vi "Get_Fluid_Properties.vi"(4 "Fluid Properties":T3) -> (1 "Thermo and Transport Properties":T1)   [LabVIEW 2011]
uses:
  fluid_types.ctl
  fluid_properties.ctl
  <vilib>/gmath/interp.llb/Create Mesh Grid (2D) (x,y arrays).vi
  <vilib>/Utility/file.llb/Read From Spreadsheet File (DBL).vi
  <vilib>/gmath/interp.llb/Interpolate 2D (2d X,Y).vi
  <vilib>/gmath/NI_Gmath.lvlib
panel:
  out "Data":dbl[][][](array[numeric])
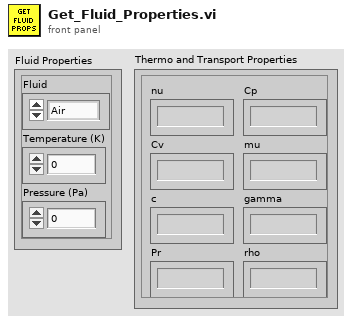
[diagram p1: front panel]
types:
  T1 = typedef "fluid_properties.ctl" = cluster{"nu":dbl, "c":dbl, "Pr":dbl, "Cp":dbl, "Cv":dbl, "gamma":dbl, "mu":dbl, "rho":dbl}
  T2 = typedef "fluid_types.ctl" = enum16{"Air", "Water"}
  T3 = cluster{"Fluid":T2, "Temperature (K)":dbl, "Pressure (Pa)":dbl}
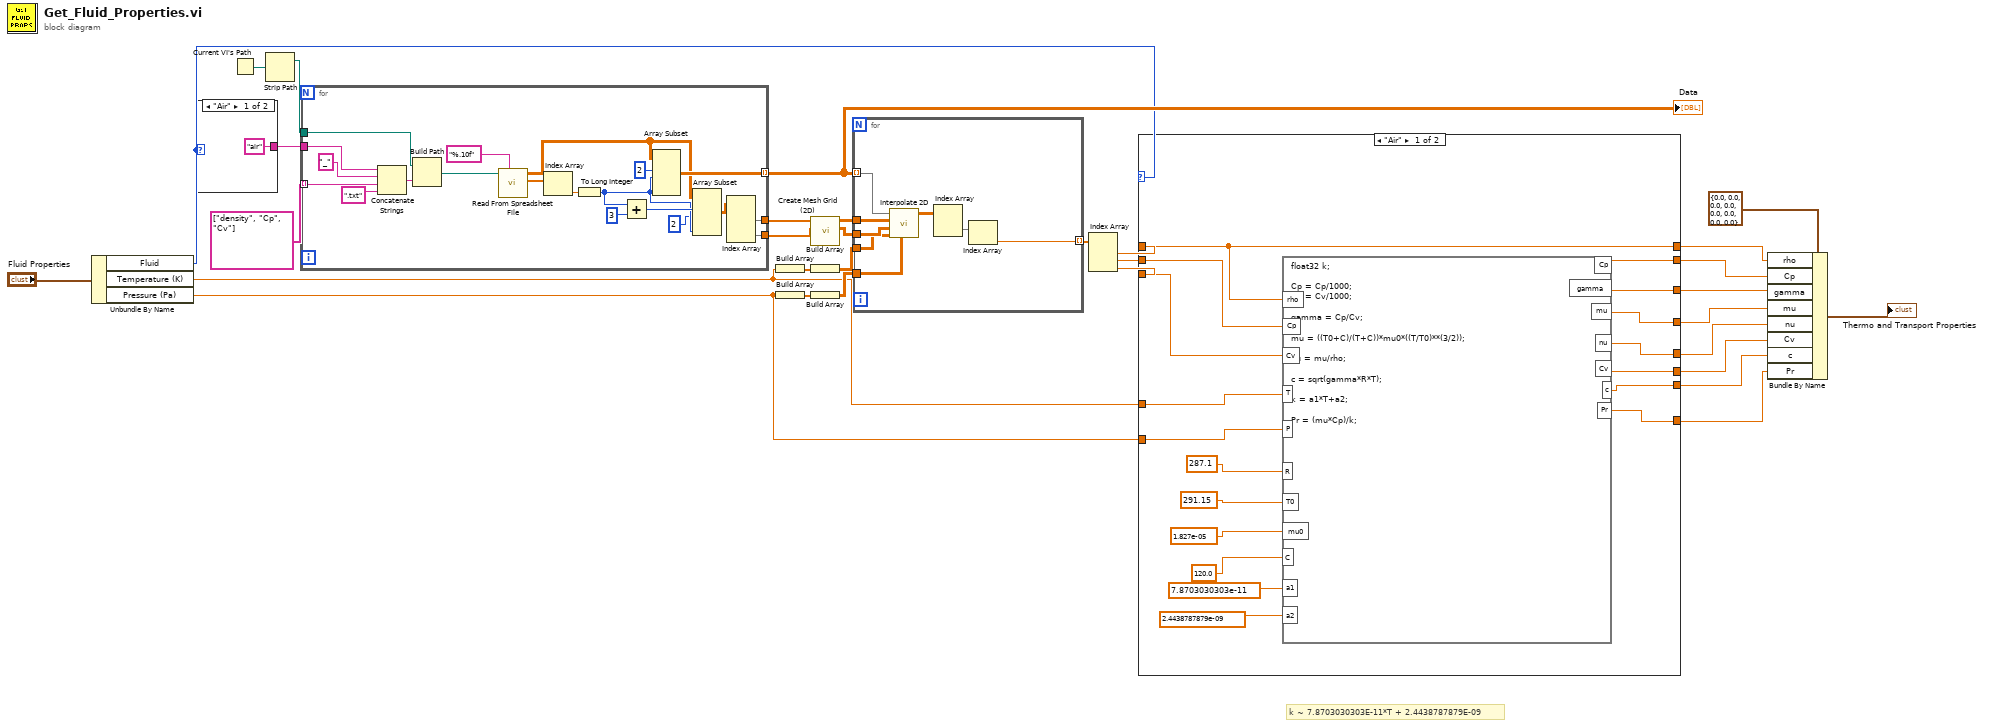
[diagram p0: block diagram]
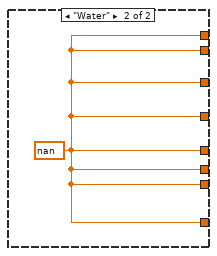
[diagram p2: hidden frame]
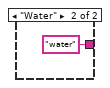
[diagram p3: hidden frame]
diagram:
  # "k ~ 7.8703030303E-11*T + 2.4438787879E-09"
  n1 = Unbundle By Name("Fluid Properties") -> ("Fluid"=w11:T2, "Temperature (K)"=w12:dbl, "Pressure (Pa)"=w13:dbl)
  n2 = case shown="\"Air\"" w11 {
    tunnel: ["air" "water"] -> w30
    frame "Air" {
    }
    frame "Water" {
    }
  }
  n3 = Current VI's Path() -> (path=w29:path)
  n4 = Strip Path(path=w29) -> (stripped path=w27:path)  [unwired: 1 out]
  n5 = for {
    tunnel: w30 -> [w52]
    tunnel: string[] ["density", "Cp", "Cv"] -> [w50] mode=indexing
    tunnel: w27 -> [w53]
    tunnel: [w44] -> w24 mode=indexing
    tunnel: [w35] -> w25
    tunnel: [w34] -> w26
    n6 = Concatenate Strings(w52, "_" ("string"), w50, ".txt" ("string")) -> (w48:string)
    n7 = Build Path(base path=w53, name or relative path=w48) -> (appended path=w47:path)
    n8 = call-poly <vilib>:"Read From Spreadsheet File.vi"("format (%.3f)"="%.10f", "file path (dialog if empty)"=w47) -> ("first row"=w45:dbl[], "all rows"=w41:dbl[][])  [unwired: 5 in, 3 out]
    n9 = Index Array(array=w45) -> (element=w43:dbl)  [unwired: 1 in]
    n10 = To Long Integer(number=w43) -> (32bit integer=w38:i32)
    n11 = Add(x=w38, y=3) -> (x+y=w39:i32)
    n12 = Array Subset(array=w41, index (row)=2 ("index"), length (row)=w38, length (col)=w38) -> (w44:dbl[][])  [unwired: 1 in]
    n13 = Array Subset(array=w41, index (row)=w39, length (row)=2 ("length"), length (col)=w38) -> (w36:dbl[][])  [unwired: 1 in]
    n14 = Index Array(array=w36) -> (element #1=w34:dbl[], element #2=w35:dbl[])  [unwired: 4 in]
  }
  "Data" <- w24
  n15 = Build Array(w12) -> (w20:dbl[])
  n16 = Build Array(w13) -> (w18:dbl[])
  n17 = call-poly <vilib>:"Create Mesh Grid (2D).vi"("y domain"=w25, "x domain"=w26) -> ("Y"=w22:dbl[][], "X"=w23:dbl[][])  [unwired: 7 in, 1 out]
  n18 = Build Array(w20) -> (w21:dbl[][])
  n19 = Build Array(w18) -> (w19:dbl[][])
  n20 = for {
    tunnel: w24 -> [w61] mode=indexing
    tunnel: w23 -> [w60]
    tunnel: w22 -> [w59]
    tunnel: w21 -> [w58]
    tunnel: w19 -> [w57]
    tunnel: [w54] -> w17 mode=indexing
    n21 = call-poly <vilib>:"Interpolate 2D.vi"("yi"=w57, "xi"=w58, "Y"=w59, "X"=w60, "Z"=w61) -> ("zi"=w56:dbl[][])  [unwired: 3 in, 3 out]
    n22 = Index Array(array=w56) -> (element=w55:dbl[])  [unwired: 2 in]
    n23 = Index Array(array=w55) -> (element=w54:dbl)  [unwired: 1 in]
  }
  n24 = Index Array(array=w17) -> (element #1=w16:dbl, element #2=w15:dbl, element #3=w14:dbl)  [unwired: 3 in]
  n25 = case shown="\"Air\"" w11 {
    tunnel: w16 -> [w66 _]
    tunnel: w15 -> [w65 _]
    tunnel: w14 -> [w64 _]
    tunnel: w13 -> [w79 _]
    tunnel: w12 -> [w78 _]
    tunnel: [w71 w80] -> w3
    tunnel: [w70 w80] -> w2
    tunnel: [w69 w80] -> w4
    tunnel: [w68 w80] -> w6
    tunnel: [w67 w80] -> w7
    tunnel: [w66 w80] -> w9
    tunnel: [w63 w80] -> w8
    tunnel: [w62 w80] -> w5
    frame "Air" {
      n26 = formula code="float32 k;\n\nCp = Cp/1000;\nCv = Cv/1000;\n\ngamma = Cp/Cv;\n\nmu = ((T0+C)/(T+C))*mu0*((T/T0)**(3/2));\n\nnu = mu/rho;\n\nc = sqrt(gamma*R*T);\n\nk = a1*T+a2;\n\nPr = (mu*Cp)/k;"("rho"=w66, "Cp"=w65, "Cv"=w64, "T"=w78, "P"=w79, "R"=287.1 ("input variable"), "T0"=291.15 ("input variable"), "mu0"=1.827e-05 ("input variable"), "C"=120.0 ("input variable"), "a1"=7.8703030303e-11 ("input variable"), "a2"=2.4438787879e-09 ("input variable")) -> ("gamma"=w71:dbl, "mu"=w70:dbl, "nu"=w69:dbl, "c"=w68:dbl, "Pr"=w67:dbl, "Cp"=w63:dbl, "Cv"=w62:dbl)
    }
    frame "Water" {
      w80 = nan
    }
  }
  n27 = Bundle By Name(cluster=T1 {"nu"=0.0, "c"=0.0, "Pr"=0.0, "Cp"=0.0, "Cv"=0.0, "gamma"=0.0, "mu"=0.0, "rho"=0.0} ("Thermo and Transport Properties 2"), "rho"=w9, "Cp"=w8, "gamma"=w3, "mu"=w2, "nu"=w4, "Cv"=w5, "c"=w6, "Pr"=w7) -> (→"Thermo and Transport Properties":T1)
